vi "10_NOV_COMMAND.vi"() -> ()   [LabVIEW 2020]
uses:
  <instrlib>/Agilent B2900 Series/Agilent B2900 Series.lvlib
panel:
  out "COMMAND":string
  in  "Measure":enum16{"Current", "Voltage", "Resistance"}(ring)
  in  "Source Voltage(V)":dbl
  in  "Channel":u16(ring) items=["", "1", "2"]
  out "Measurement":dbl
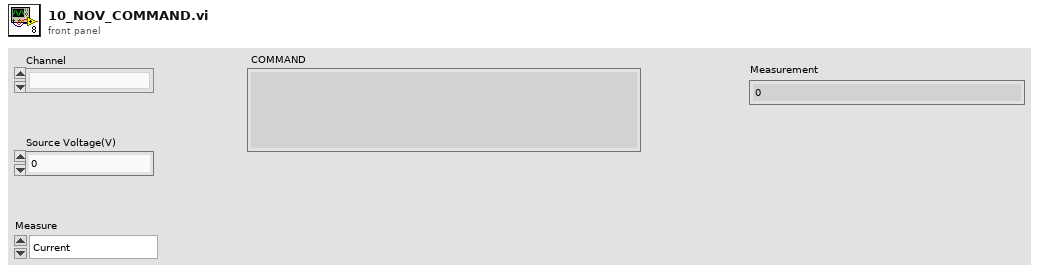
[diagram p1: front panel]
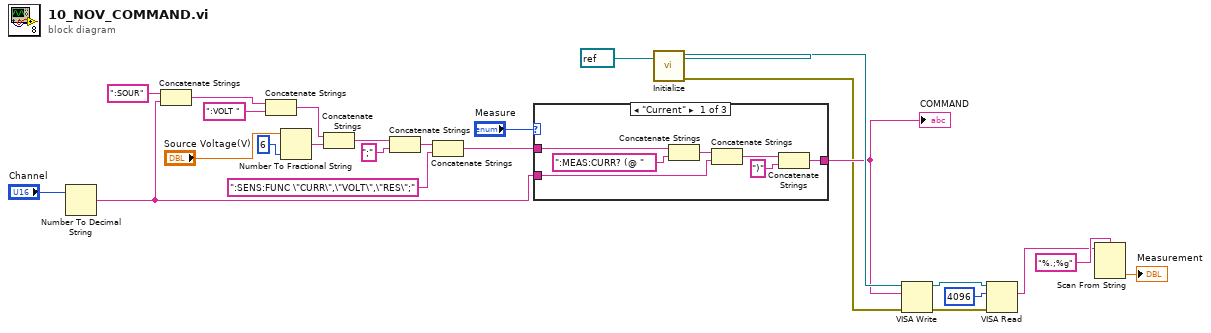
[diagram p0: block diagram]
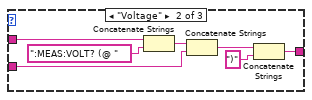
[diagram p2: hidden frame]
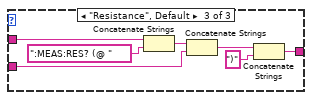
[diagram p3: hidden frame]
diagram:
  n1 = Number To Decimal String(number="Channel") -> (decimal integer string=w4:string)  [unwired: 1 in]
  n2 = Concatenate Strings(":SOUR", w4) -> (w16:string)
  n3 = Concatenate Strings(w16, ":VOLT ") -> (w14:string)
  n4 = Number To Fractional String(number="Source Voltage(V)", precision (6)=i16 6) -> (F-format string=w9:string)  [unwired: 2 in]
  n5 = Concatenate Strings(w14, w9) -> (w13:string)
  n6 = Concatenate Strings(w13, ";" ("string")) -> (w8:string)
  n7 = Concatenate Strings(w8, ":SENS:FUNC \"CURR\",\"VOLT\",\"RES\";") -> (w5:string)
  n8 = case shown="\"Current\"" "Measure" {
    tunnel: w5 -> [w28 w39 w42]
    tunnel: w4 -> [w27 w36 w41]
    tunnel: [w26 w33 w40] -> w3
    frame "Current" {
      n9 = Concatenate Strings(w28, ":MEAS:CURR? (@ " ("string")) -> (w31:string)
      n10 = Concatenate Strings(w31, w27) -> (w30:string)
      n11 = Concatenate Strings(w30, ")" ("string")) -> (w26:string)
    }
    frame "Voltage" {
      n12 = Concatenate Strings(w39, ":MEAS:VOLT? (@ " ("string")) -> (w37:string)
      n13 = Concatenate Strings(w37, w36) -> (w35:string)
      n14 = Concatenate Strings(w35, ")" ("string")) -> (w33:string)
    }
    frame "Resistance", Default {
      n15 = Concatenate Strings(w42, ":MEAS:RES? (@ " ("string")) -> (w45:string)
      n16 = Concatenate Strings(w45, w41) -> (w44:string)
      n17 = Concatenate Strings(w44, ")" ("string")) -> (w40:string)
    }
  }
  "COMMAND" <- w3
  n18 = call <instrlib>:"Initialize.vi"("VISA resource name"=refnum<visa-resource-name> "USB0::0x0957::0x8E18::MY51140695::INSTR") -> ("error out"=w2:errorcluster, "VISA resource name out"=w21:refnum<visa-resource-name>)  [unwired: 9 in]
  n19 = VISA Write(VISA resource name=w21, write buffer=w3, error in (no error)=w2) -> (VISA resource name out=w24:refnum<visa-resource-name>, error out=w23:errorcluster)  [unwired: 1 out]
  n20 = VISA Read(VISA resource name=w24, byte count=u32 4096, error in (no error)=w23) -> (read buffer=w18:string)  [unwired: 3 out]
  n21 = Scan From String(format string="%.;%g", input string=w18) -> (output 1=→"Measurement":dbl)  [unwired: 3 in, 3 out]
